vi "Compare Sizesv1.vi"(2 "Below Area":dbl, 3 "First  Area":dbl, 4 "Above Area":dbl) -> (0 "Closest Area":dbl, 1 "Above?":bool)   [LabVIEW 2013]
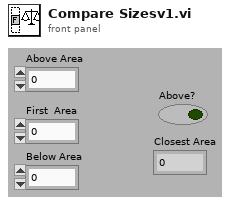
[diagram p1: front panel]
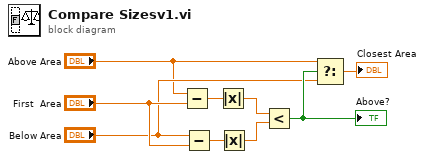
[diagram p0: block diagram]
diagram:
  n1 = Subtract(x="Above Area", y="First  Area") -> (x-y=w4:dbl)
  n2 = Subtract(x="Below Area", y="First  Area") -> (x-y=w3:dbl)
  n3 = Absolute Value(x=w4) -> (abs(x)=w2:dbl)
  n4 = Absolute Value(x=w3) -> (abs(x)=w1:dbl)
  n5 = Less?(x=w2, y=w1) -> (x < y?=w9:bool)
  "Above?" <- w9
  n6 = Select(t="Above Area", s=w9, f="Below Area") -> (s? t:f=→"Closest Area":dbl)
